vi "Write.vi"(8 "error in (no error)":errorcluster, 9 "Start address":string, 10 "Read Type":variant, 11 "MelsecTCP in":refnum<class "InovanceSerialModbusRtu.lvclass">) -> (0 "error out":errorcluster, 3 "MelsecTCP out":refnum<class "InovanceSerialModbusRtu.lvclass">)   [LabVIEW 2020, in "HslCommunication.lvlib" / "InovanceSerialModbusRtu.lvclass"]
uses:
  InovanceSerialModbusRtu.lvclass
  D:/Git/Labview-Libraries/Libraries/HslCommunication/Abstract PLC Controler/Abstract PLC Controler.lvclass
  EventLogger.lvlibp/1abvi3w/vi.lib/gpm_packages/@cs/event-logger/Source/Composed Log/Types/Log Level.ctl
  Abstract PLC Controler/Abstract PLC Controler.lvclass/Abstract PLC Controler.ctl
  D:/Git/Labview-Libraries/Libraries/HslCommunication/_Dependenciecs/HslCommunication.dll
  _Dependenciecs/HslCommunication.dll
  Read reference.vi
  Abstract PLC Controler/Abstract PLC Controler.lvclass
  <vilib>/Utility/Data Type/NI_Data Type.lvlib
  EventLogger.lvlibp/Logger.lvclass
  EventLogger.lvlibp/1abvi3w/vi.lib/gpm_packages/@cs/event-logger/Source/Composed Log/Composed Log.lvlib
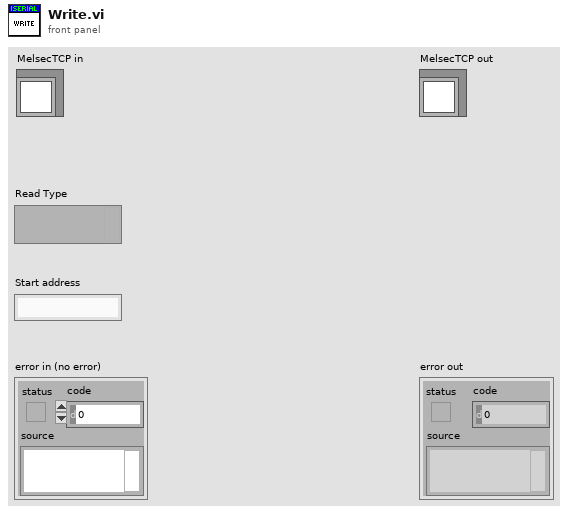
[diagram p1: front panel]
types:
  T1 = typedef "EventLogger.lvlibp/Composed Log.lvlib/Log Level.ctl" = enum16{"Debug", "Info", "Warning", "Error", "Critical"}
  T2 = typedef "NI_Data Type.lvlib/Data Type.ctl" = enum8{"Invalid Type", "Void", "I8", "I16", "I32", "I64", "U8", "U16", "U32", "U64", "Single Float", "Double Float", "Extended Float", "Single Complex", "Double Complex", "Extended Complex", "Enum U8", "Enum U16", "Enum U32", "Enum U64", "Single Float With Unit", "Double Float With Unit", "Extended Float With Unit", "Single Complex with Unit", "Double Complex with Unit", "Extended Complex with Unit", "Boolean", "String", "Path", "Picture", "Tag", "Array", "Cluster", "Variant", "LV Variant", "Waveform", "Timestamp", "Digital Waveform", "Digital Data", "ExpressData", "Refnum", "External Data", "VI", "Poly VI", "LabVIEW Class Instance", "Fixed Point", "Set Collection", "Map Collection"}
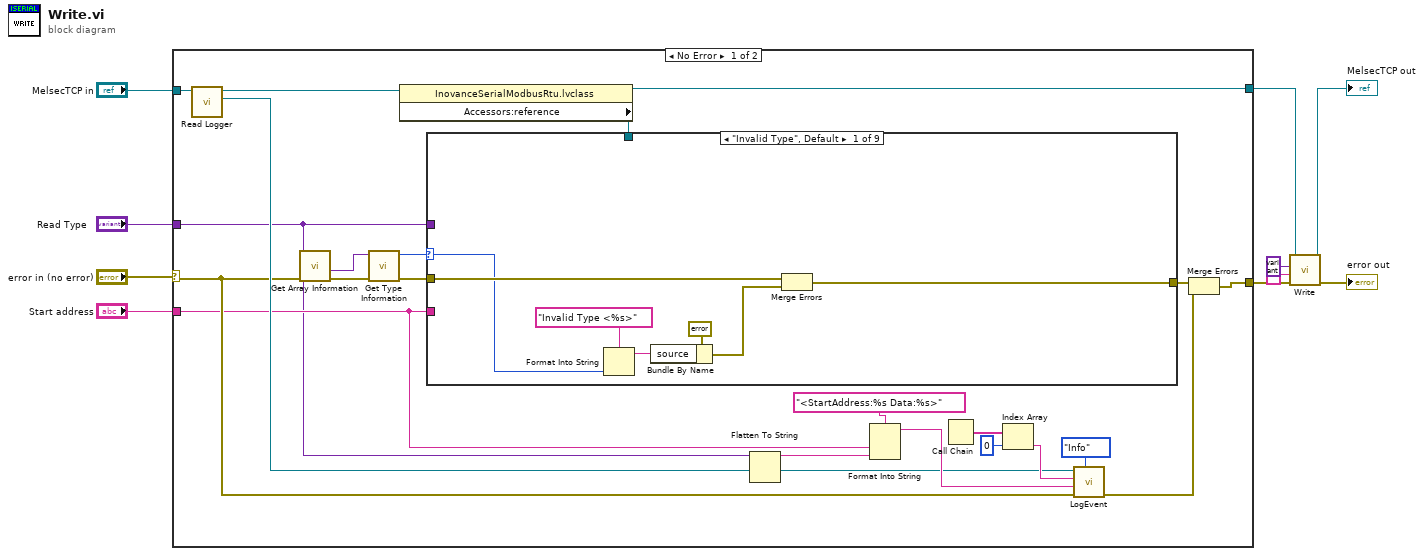
[diagram p0: block diagram]
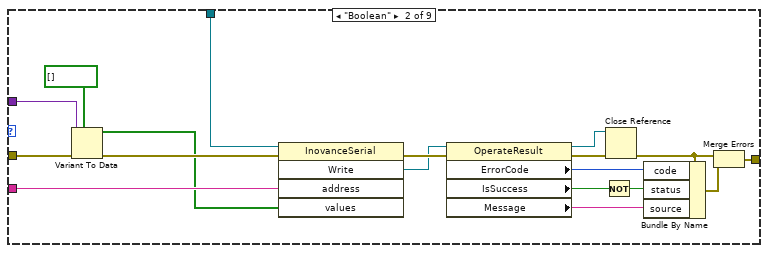
[diagram p2: hidden frame]
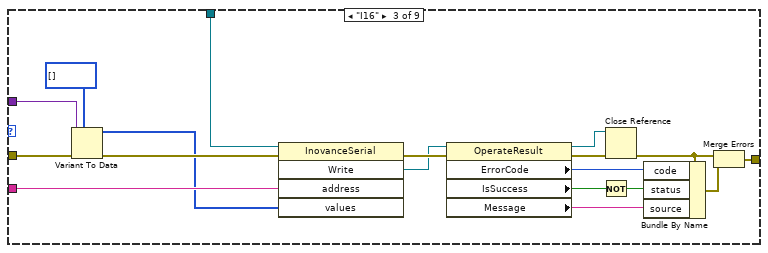
[diagram p3: hidden frame]
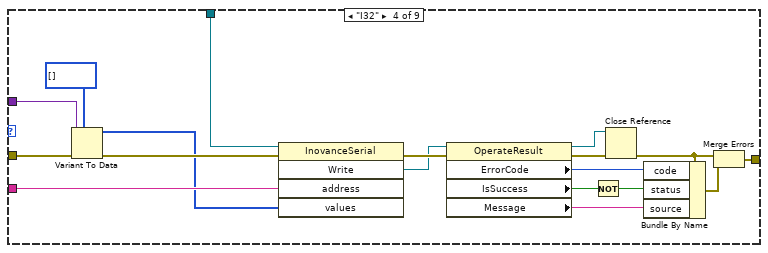
[diagram p4: hidden frame]
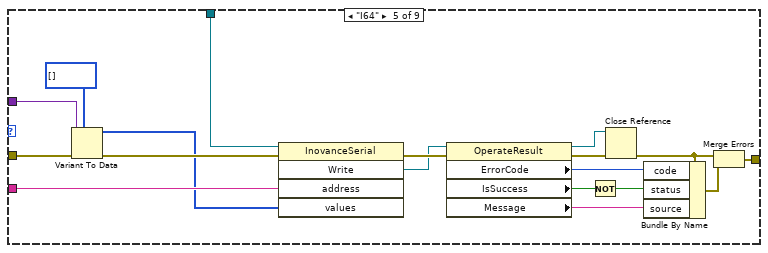
[diagram p5: hidden frame]
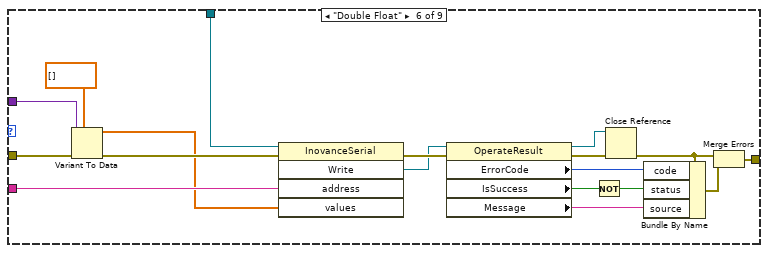
[diagram p6: hidden frame]
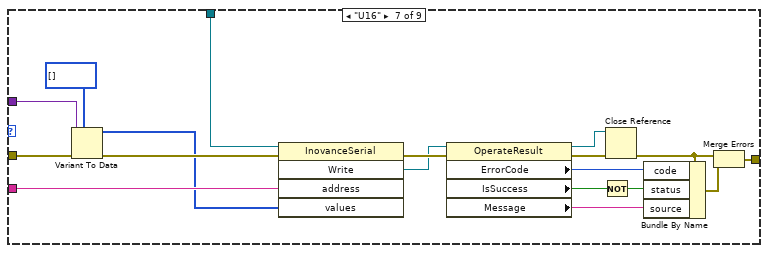
[diagram p7: hidden frame]
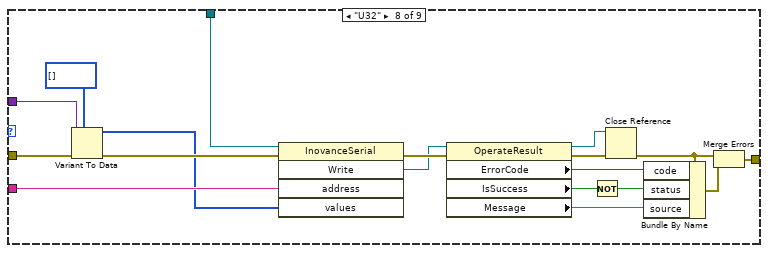
[diagram p8: hidden frame]
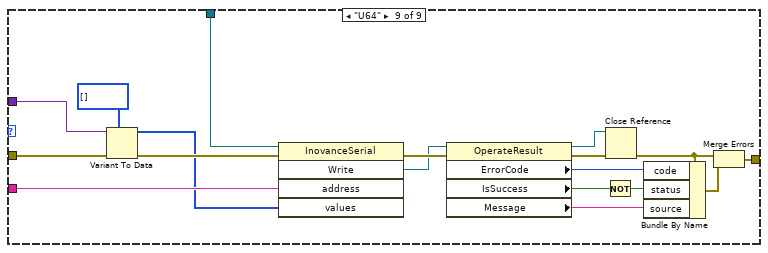
[diagram p9: hidden frame]
diagram:
  n1 = case shown="No Error" "error in (no error)" {
    selector: "error in (no error)" -> [w16 w185]
    tunnel: "MelsecTCP in" -> [w32 w184]
    tunnel: [w29 w184] -> w4
    tunnel: "Start address" -> [w15 _]
    tunnel: [w12 w185] -> w7
    tunnel: "Read Type" -> [w14 _]
    frame No Error {
      n2 = call "Read Logger.vi"("Abstract PLC Controler in"=w32) -> ("EventLogger.lvlibp:Logger.lvclass"=w17:refnum<class "Logger.lvclass">, "Abstract PLC Controler out"=w18:refnum<class "InovanceSerialModbusRtu.lvclass">)  [unwired: 9 in]
      n3 = call <vilib>:"Get Array Information.vi"("error in (no error)"=w16, "variant"=w14) -> ("error out"=w27:errorcluster, "array element data type"=w28:variant)  [unwired: 6 in, 2 out]
      n4 = call <vilib>:"Get Type Information.vi"("error in (no error)"=w27, "variant"=w28) -> ("error out"=w26:errorcluster, "type"=w25:T2)  [unwired: 5 in, 3 out]
      n5 = property class="InovanceSerialModbusRtu.lvclass"(reference=w18) -> (reference out=w29:refnum<class "InovanceSerialModbusRtu.lvclass">, "Accessors:reference"=w31:refnum<k24>)  [unwired: 1 in, 1 out]
      n6 = case shown="\"Invalid Type\", Default" w25 {
        selector: w25 -> [w37 _ _ _ _ _ _ _ _]
        tunnel: w31 -> [_ w57 w75 w93 w111 w129 w147 w165 w183]
        tunnel: w15 -> [_ w56 w74 w92 w110 w128 w146 w164 w182]
        tunnel: [w38 w55 w73 w91 w109 w127 w145 w163 w181] -> w30
        tunnel: w14 -> [_ w49 w67 w85 w103 w121 w139 w157 w175]
        tunnel: w26 -> [w39 w48 w66 w84 w102 w120 w138 w156 w174]
        frame "Invalid Type", Default {
          n7 = Format Into String(format string="Invalid Type <%s>", w37) -> (resulting string=w34:string)  [unwired: 2 in, 1 out]
          n8 = Bundle By Name(cluster=errorcluster {"status"=TRUE, "code"=-1, "source"=""} ("error IO"), "source"=w34) -> (w33:errorcluster)
          n9 = Merge Errors(w39, w33) -> (w38:errorcluster)
        }
        frame "Boolean" {
          n10 = Variant To Data(error in=w48, type=bool[] [], Variant=w49) -> (data=w41:bool[], error out=w43:errorcluster)
          n11 = invoke class="InovanceSerial" method="Write"(reference=w57, error in=w43, "address"=w56, "values"=w41) -> (error out=w47:errorcluster, "Write"=w45:refnum<k24>)  [unwired: 1 in, 3 out]
          n12 = property class="OperateResult"(reference=w45, error in=w47) -> (reference out=w44:refnum<k24>, error out=w46:errorcluster, "ErrorCode"=w54:i32, "IsSuccess"=w53:bool, "Message"=w52:string)
          n13 = Not(x=w53) -> (.not. x?=w40:bool)
          n14 = Close Reference(reference=w44, error in (no error)=w46) -> (error out=w51:errorcluster)
          n15 = Bundle By Name(cluster=w51, "code"=w54, "status"=w40, "source"=w52) -> (w50:errorcluster)
          n16 = Merge Errors(w51, w50) -> (w55:errorcluster)
        }
        frame "I16" {
          n17 = Variant To Data(error in=w66, type=i16[] [], Variant=w67) -> (data=w59:i16[], error out=w61:errorcluster)
          n18 = invoke class="InovanceSerial" method="Write"(reference=w75, error in=w61, "address"=w74, "values"=w59) -> (error out=w65:errorcluster, "Write"=w63:refnum<k24>)  [unwired: 1 in, 3 out]
          n19 = property class="OperateResult"(reference=w63, error in=w65) -> (reference out=w62:refnum<k24>, error out=w64:errorcluster, "ErrorCode"=w72:i32, "IsSuccess"=w71:bool, "Message"=w70:string)
          n20 = Not(x=w71) -> (.not. x?=w58:bool)
          n21 = Close Reference(reference=w62, error in (no error)=w64) -> (error out=w69:errorcluster)
          n22 = Bundle By Name(cluster=w69, "code"=w72, "status"=w58, "source"=w70) -> (w68:errorcluster)
          n23 = Merge Errors(w69, w68) -> (w73:errorcluster)
        }
        frame "I32" {
          n24 = Variant To Data(error in=w84, type=i32[] [], Variant=w85) -> (data=w77:i32[], error out=w79:errorcluster)
          n25 = invoke class="InovanceSerial" method="Write"(reference=w93, error in=w79, "address"=w92, "values"=w77) -> (error out=w83:errorcluster, "Write"=w81:refnum<k24>)  [unwired: 1 in, 3 out]
          n26 = property class="OperateResult"(reference=w81, error in=w83) -> (reference out=w80:refnum<k24>, error out=w82:errorcluster, "ErrorCode"=w90:i32, "IsSuccess"=w89:bool, "Message"=w88:string)
          n27 = Not(x=w89) -> (.not. x?=w76:bool)
          n28 = Close Reference(reference=w80, error in (no error)=w82) -> (error out=w87:errorcluster)
          n29 = Bundle By Name(cluster=w87, "code"=w90, "status"=w76, "source"=w88) -> (w86:errorcluster)
          n30 = Merge Errors(w87, w86) -> (w91:errorcluster)
        }
        frame "I64" {
          n31 = Variant To Data(error in=w102, type=i64[] [], Variant=w103) -> (data=w95:i64[], error out=w97:errorcluster)
          n32 = invoke class="InovanceSerial" method="Write"(reference=w111, error in=w97, "address"=w110, "values"=w95) -> (error out=w101:errorcluster, "Write"=w99:refnum<k24>)  [unwired: 1 in, 3 out]
          n33 = property class="OperateResult"(reference=w99, error in=w101) -> (reference out=w98:refnum<k24>, error out=w100:errorcluster, "ErrorCode"=w108:i32, "IsSuccess"=w107:bool, "Message"=w106:string)
          n34 = Not(x=w107) -> (.not. x?=w94:bool)
          n35 = Close Reference(reference=w98, error in (no error)=w100) -> (error out=w105:errorcluster)
          n36 = Bundle By Name(cluster=w105, "code"=w108, "status"=w94, "source"=w106) -> (w104:errorcluster)
          n37 = Merge Errors(w105, w104) -> (w109:errorcluster)
        }
        frame "Double Float" {
          n38 = Variant To Data(error in=w120, type=dbl[] [], Variant=w121) -> (data=w113:dbl[], error out=w115:errorcluster)
          n39 = invoke class="InovanceSerial" method="Write"(reference=w129, error in=w115, "address"=w128, "values"=w113) -> (error out=w119:errorcluster, "Write"=w117:refnum<k24>)  [unwired: 1 in, 3 out]
          n40 = property class="OperateResult"(reference=w117, error in=w119) -> (reference out=w116:refnum<k24>, error out=w118:errorcluster, "ErrorCode"=w126:i32, "IsSuccess"=w125:bool, "Message"=w124:string)
          n41 = Not(x=w125) -> (.not. x?=w112:bool)
          n42 = Close Reference(reference=w116, error in (no error)=w118) -> (error out=w123:errorcluster)
          n43 = Bundle By Name(cluster=w123, "code"=w126, "status"=w112, "source"=w124) -> (w122:errorcluster)
          n44 = Merge Errors(w123, w122) -> (w127:errorcluster)
        }
        frame "U16" {
          n45 = Variant To Data(error in=w138, type=u16[] [], Variant=w139) -> (data=w131:u16[], error out=w133:errorcluster)
          n46 = invoke class="InovanceSerial" method="Write"(reference=w147, error in=w133, "address"=w146, "values"=w131) -> (error out=w137:errorcluster, "Write"=w135:refnum<k24>)  [unwired: 1 in, 3 out]
          n47 = property class="OperateResult"(reference=w135, error in=w137) -> (reference out=w134:refnum<k24>, error out=w136:errorcluster, "ErrorCode"=w144:i32, "IsSuccess"=w143:bool, "Message"=w142:string)
          n48 = Not(x=w143) -> (.not. x?=w130:bool)
          n49 = Close Reference(reference=w134, error in (no error)=w136) -> (error out=w141:errorcluster)
          n50 = Bundle By Name(cluster=w141, "code"=w144, "status"=w130, "source"=w142) -> (w140:errorcluster)
          n51 = Merge Errors(w141, w140) -> (w145:errorcluster)
        }
        frame "U32" {
          n52 = Variant To Data(error in=w156, type=u32[] [], Variant=w157) -> (data=w149:u32[], error out=w151:errorcluster)
          n53 = invoke class="InovanceSerial" method="Write"(reference=w165, error in=w151, "address"=w164, "values"=w149) -> (error out=w155:errorcluster, "Write"=w153:refnum<k24>)  [unwired: 1 in, 3 out]
          n54 = property class="OperateResult"(reference=w153, error in=w155) -> (reference out=w152:refnum<k24>, error out=w154:errorcluster, "ErrorCode"=w162:i32, "IsSuccess"=w161:bool, "Message"=w160:string)
          n55 = Not(x=w161) -> (.not. x?=w148:bool)
          n56 = Close Reference(reference=w152, error in (no error)=w154) -> (error out=w159:errorcluster)
          n57 = Bundle By Name(cluster=w159, "code"=w162, "status"=w148, "source"=w160) -> (w158:errorcluster)
          n58 = Merge Errors(w159, w158) -> (w163:errorcluster)
        }
        frame "U64" {
          n59 = Variant To Data(error in=w174, type=u64[] [], Variant=w175) -> (data=w167:u64[], error out=w169:errorcluster)
          n60 = invoke class="InovanceSerial" method="Write"(reference=w183, error in=w169, "address"=w182, "values"=w167) -> (error out=w173:errorcluster, "Write"=w171:refnum<k24>)  [unwired: 1 in, 3 out]
          n61 = property class="OperateResult"(reference=w171, error in=w173) -> (reference out=w170:refnum<k24>, error out=w172:errorcluster, "ErrorCode"=w180:i32, "IsSuccess"=w179:bool, "Message"=w178:string)
          n62 = Not(x=w179) -> (.not. x?=w166:bool)
          n63 = Close Reference(reference=w170, error in (no error)=w172) -> (error out=w177:errorcluster)
          n64 = Bundle By Name(cluster=w177, "code"=w180, "status"=w166, "source"=w178) -> (w176:errorcluster)
          n65 = Merge Errors(w177, w176) -> (w181:errorcluster)
        }
      }
      n66 = Flatten To String(anything=w14) -> (data string=w13:string)  [unwired: 3 in, 2 out]
      n67 = Format Into String(format string="<StartAddress:%s Data:%s>", w15, w13) -> (resulting string=w21:string)  [unwired: 2 in, 1 out]
      n68 = Call Chain() -> (call chain=w24:string[])
      n69 = Index Array(array=w24, index=0) -> (element=w20:string)
      n70 = call "LogEvent.vi"("Event Level"=Log_Level."Info", "error in (no error)"=w16, "Data To Log"=w21, "SourceID"=w20, "Logger in"=w17) -> ("error out"=w11:errorcluster)  [unwired: 5 in, 1 out]
      n71 = Merge Errors(w30, w11) -> (w12:errorcluster)
    }
    frame Error {
    }
  }
  n72 = call-parent "Write.vi"("error in (no error)"=w7, "Start address"="", "Read Type"=variant, "MelsecTCP in"=w4) -> ("error out"=→"error out":errorcluster, "MelsecTCP out"=→"MelsecTCP out":refnum<class "InovanceSerialModbusRtu.lvclass">)  [unwired: 6 in]
